vi "Build Result Cluster.vi"(8 "error in (no error)":errorcluster, 9 "Pass?":bool, 10 "Actual Value":variant, 11 "Action Step in":refnum<class "Action Step.lvclass">) -> (0 "error out":errorcluster, 2 "Result":T1, 3 "Action Step out":refnum<class "Action Step.lvclass">)   [LabVIEW 2020, in "MacroAssert.lvlib" / "Action Step.lvclass"]
doc: "Builds a result cluster from the given step, <B>Actual Value</B>, and <B>Pass?</B>."
uses:
  Action Step.lvclass
  Action Step.lvclass/Action Step.ctl
  CTLs/Result.ctl
  MacroAssert.lvlib
  CTLs/Report Data.ctl
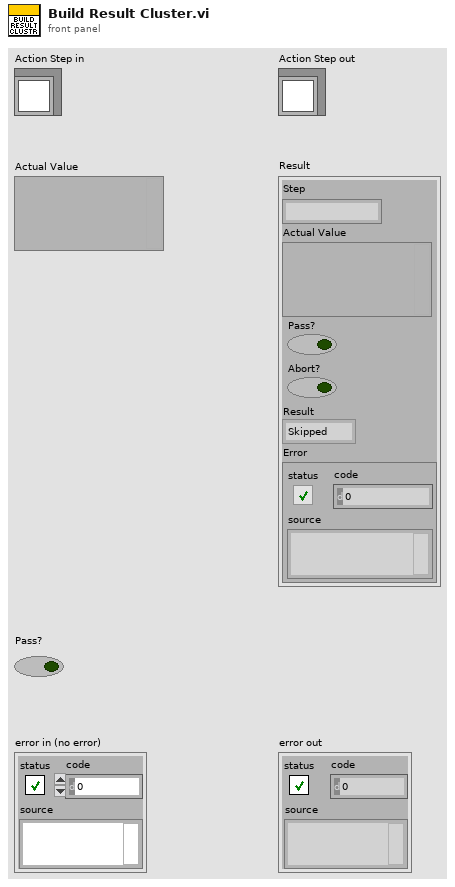
[diagram p1: front panel]
types:
  T1 = typedef "MacroAssert.lvlib/Report Data.ctl" = cluster{"Step":string, "Actual Value":variant, "Pass?":bool, "Abort?":bool, "Result":T2, "Error":errorcluster}
  T2 = typedef "MacroAssert.lvlib/Result.ctl" = enum16{"Skipped", "Pass", "Fail", "Complete", "Error"}
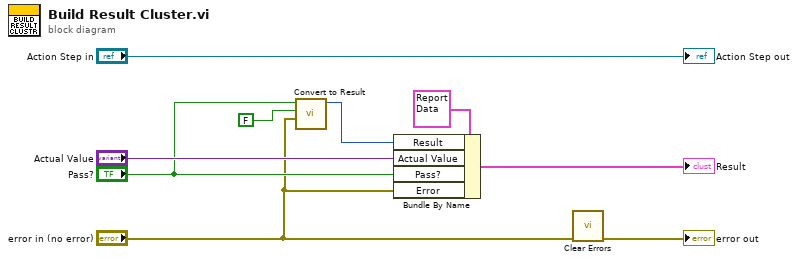
[diagram p0: block diagram]
diagram:
  n1 = call "Convert to Result.vi"("Error"="error in (no error)", "Is Assertion?"=FALSE, "Pass?"="Pass?") -> ("Result"=w1:T2)  [unwired: 8 in]
  n2 = Bundle By Name(cluster=T1 {"Step"="", "Actual Value"=variant, "Pass?"=FALSE, "Abort?"=FALSE, "Result"=enum."Skipped", "Error"={"status"=FALSE, "code"=0, "source"=""}} ("Report Data"), "Result"=w1, "Actual Value"="Actual Value", "Pass?"="Pass?", "Error"="error in (no error)") -> (→"Result":T1)
  n3 = call <vilib>:"Clear Errors.vi"("error in (no error)"="error in (no error)") -> ("error out"=→"error out":errorcluster)  [unwired: 5 in, 1 out]
  "Action Step out" <- "Action Step in"
